vi "Configure_Filters.vi"(7 "I2C Channel":u8, 8 "error in (no error)":errorcluster, 9 "Filtered Data Selection":T1(ring), 10 "High-Pass Cutoff Frequency":T2(ring), 11 "LINX Resource In":T3) -> (0 "error out":errorcluster, 3 "LINX Resource Out":T3)   [LabVIEW 2014, in "LMH-LINX.lvlib" / "LIS331HH.lvlib"]
doc: "This VI ebales and configures High-Pass output filters and Enables/Disables Filter bypass. \nLow Pass filters and cutoff frequency is based of Output Data Rate (ORD) set with Initialize.vi and Set_ODR.vi\n\n**Author: Stas Legedza"
uses:
  <vilib>/MakerHub/LINX/Public/Sensors/Accelerometer/LIS331HH/LIS331HH.lvlib
  <vilib>/MakerHub/LINX/Private/Type Defs/LINX Ref.ctl
  <vilib>/MakerHub/LINX/Private/Type Defs/Platform.ctl
  <vilib>/MakerHub/LINX/Private/Type Defs/Interface.ctl
  <vilib>/MakerHub/LINX/Private/Device/Type Defs/LINX Device Config.ctl
  <vilib>/MakerHub/LINX/Private/Device/Type Defs/TCP Config.ctl
  <vilib>/MakerHub/LINX/Private/Device/Type Defs/Channels.ctl
  <vilib>/MakerHub/LINX/Private/Local IO/LinxI2cWrite.vi
  <vilib>/MakerHub/LINX/Public/Utilities/Check Channel.vi
  <vilib>/MakerHub/LINX/Private/Utilties/Generate Error.vi
  <vilib>/MakerHub/LINX/LMH-LINX.lvlib
  <vilib>/MakerHub/LINX/Private/Device/Device.lvlib
panel:
  # "NOTE: LP Cutoff is based on a Output \nData Rate (ODR) settings\ni.e. @ODR of 50 Hz, LP_cutoff  is 37 Hz"
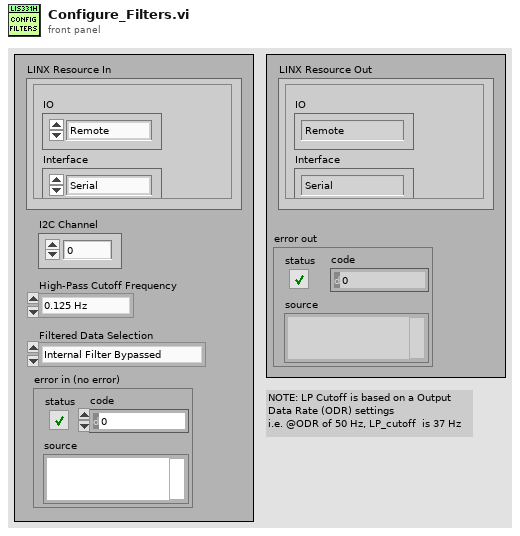
[diagram p1: front panel]
types:
  T1 = enum16{"Internal Filter Bypassed", "Data via Internal Filter"}
  T2 = enum16{"0.125 Hz", "0.25 Hz", "0.5 Hz", "1 Hz", "2 Hz", "2.5 Hz", "4 Hz", "5 Hz", "8 Hz", "10 Hz", "20 Hz"}
  T3 = typedef "LMH-LINX.lvlib/LINX Ref.ctl" = cluster{"IO":T4, "Interface":T5, "LINX Device Config":T6}
  T4 = typedef "LMH-LINX.lvlib/Platform.ctl" = enum16{"Remote", "Local"}
  T5 = typedef "LMH-LINX.lvlib/Interface.ctl" = enum16{"Serial", "TCP"}
  T6 = typedef "LMH-LINX.lvlib/Device.lvlib/LINX Device Config.ctl" = cluster{"Interface":T5, "COM Port":refnum<visa-resource-name>, "TCP Configuration":T7, "Device Family":u8, "Device ID":u8, "Device Name":string, "TCP Ref":refnum<k5>, "Channels":T8}
  T7 = typedef "LMH-LINX.lvlib/Device.lvlib/TCP Config.ctl" = cluster{"IP Address":string, "Port":u16}
  T8 = typedef "LMH-LINX.lvlib/Channels.ctl" = cluster{"DI":u8[], "DO":u8[], "AI":u8[], "AO":u8[], "PWM":u8[], "QE":u8[], "UART":u8[], "I2C 2":u8[], "SPI":u8[], "CAN":u8[], "Servo":u8[], "AI Ref (V)":dbl, "AI Resolution (Bits)":u8, "AO Ref (V)":dbl, "AO Resolution (Bits)":u8}
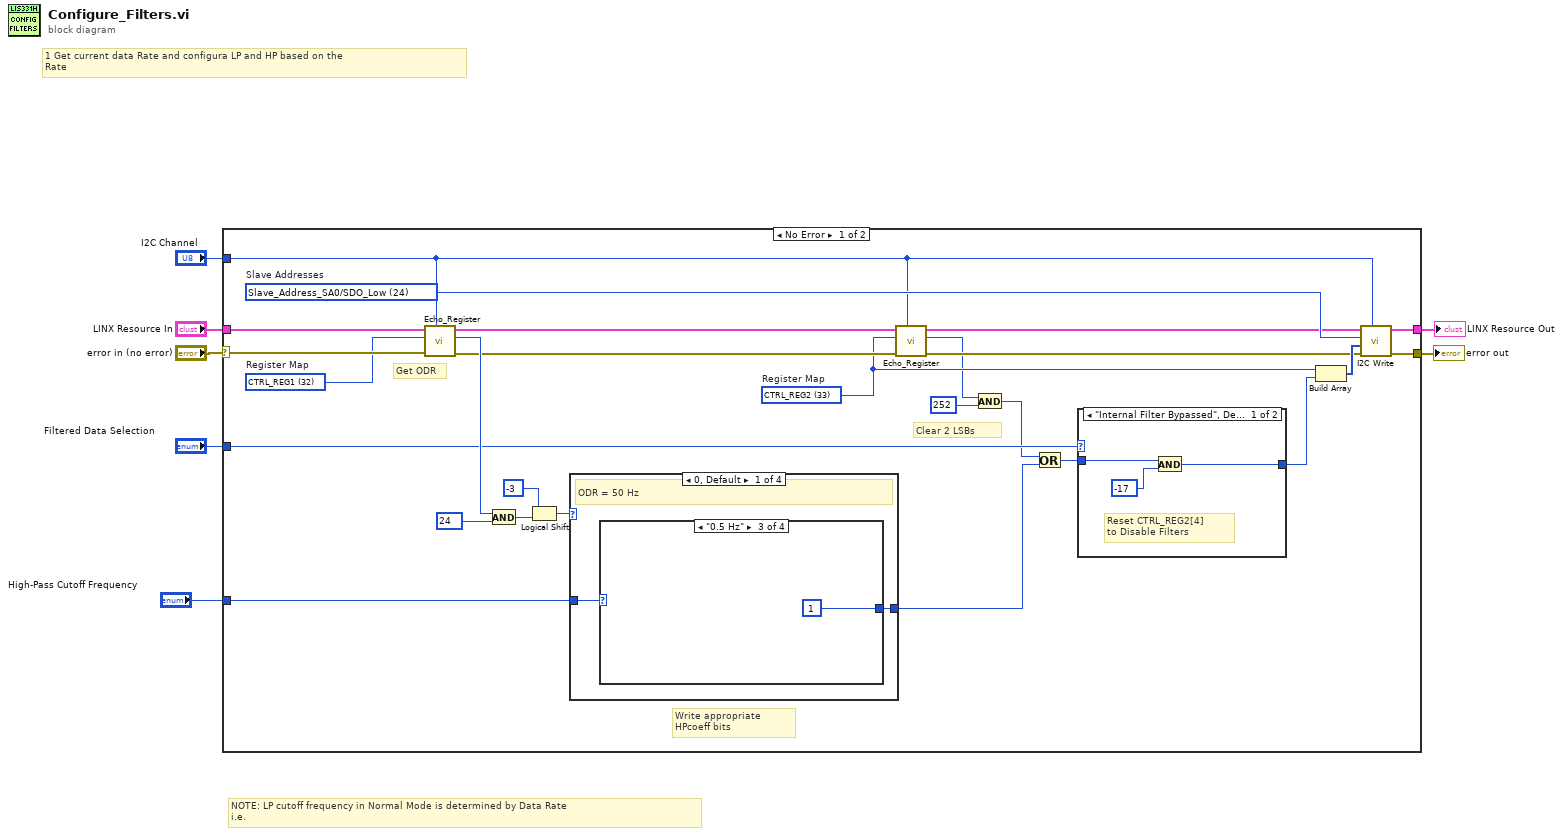
[diagram p0: block diagram]
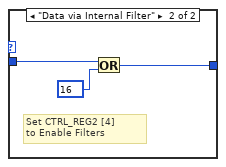
[diagram p2: hidden frame]
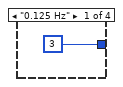
[diagram p3: hidden frame]
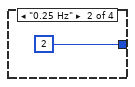
[diagram p4: hidden frame]
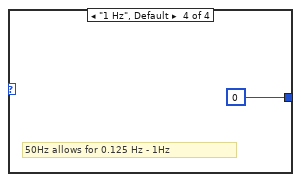
[diagram p5: hidden frame]
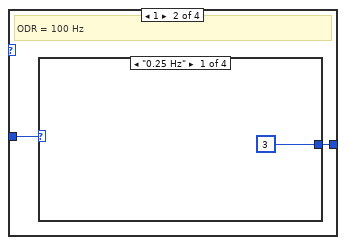
[diagram p6: hidden frame]
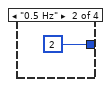
[diagram p7: hidden frame]
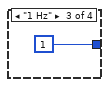
[diagram p8: hidden frame]
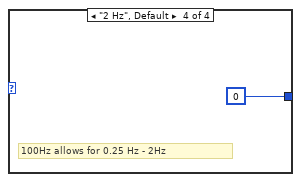
[diagram p9: hidden frame]
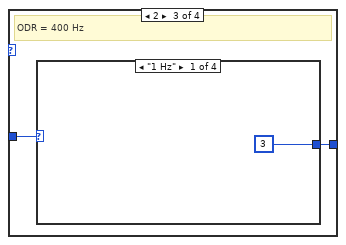
[diagram p10: hidden frame]
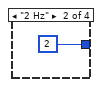
[diagram p11: hidden frame]
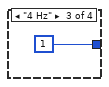
[diagram p12: hidden frame]
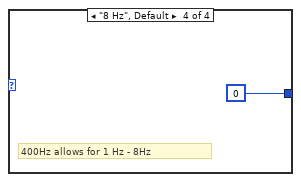
[diagram p13: hidden frame]
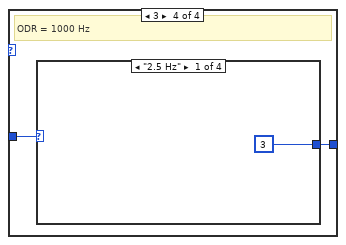
[diagram p14: hidden frame]
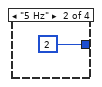
[diagram p15: hidden frame]
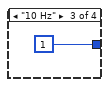
[diagram p16: hidden frame]
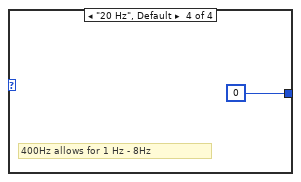
[diagram p17: hidden frame]
diagram:
  # "NOTE: LP cutoff frequency in Normal Mode is determined by Data Rate\ni.e."
  # "1 Get current data Rate and configura LP and HP based on the\nRate"
  n1 = case shown="No Error" "error in (no error)" {
    selector: "error in (no error)" -> [w29 w65]
    tunnel: [w32 w65] -> w6
    tunnel: "LINX Resource In" -> [w30 w64]
    tunnel: "I2C Channel" -> [w22 _]
    tunnel: [w31 w64] -> w3
    tunnel: "High-Pass Cutoff Frequency" -> [w25 _]
    tunnel: "Filtered Data Selection" -> [w12 _]
    frame No Error {
      w19 = u8 33 items=["CTRL_REG1"=32, "CTRL_REG2"=33, "CTRL_REG3"=34, "CTRL_REG4"=35, "CTRL_REG5"=36, "HP_FILTER_RESET"=37, "REFERENCE"=38, "STATUS_REG"=39, "OUT_X_L"=40, "OUT_X_H"=41, "OUT_Y_L"=42, "OUT_Y_H"=43, "OUT_Z_L"=44, "OUT_Z_H"=45, "INT1_CFG"=48, "INT1_SOURCE"=49, "INT1_THS"=50, "INT1_DURATION"=51, "INT2_CFG"=52, "INT2_SOURCE"=53, "INT2_THS"=54, "INT2_DURATION"=55]  # Register Map
      w18 = u8 32 items=["CTRL_REG1"=32, "CTRL_REG2"=33, "CTRL_REG3"=34, "CTRL_REG4"=35, "CTRL_REG5"=36, "HP_FILTER_RESET"=37, "REFERENCE"=38, "STATUS_REG"=39, "OUT_X_L"=40, "OUT_X_H"=41, "OUT_Y_L"=42, "OUT_Y_H"=43, "OUT_Z_L"=44, "OUT_Z_H"=45, "INT1_CFG"=48, "INT1_SOURCE"=49, "INT1_THS"=50, "INT1_DURATION"=51, "INT2_CFG"=52, "INT2_SOURCE"=53, "INT2_THS"=54, "INT2_DURATION"=55]  # Register Map
      w33 = u8 24 items=["Slave_Address_SA0/SDO_Low"=24, "Slave_Address_SA0/SDO_High"=25]  # Slave Addresses
      # "Write appropriate\nHPcoeff bits"
      # "Clear 2 LSBs"
      # "Get ODR"
      n2 = call <vilib>:"Echo_Register.vi"("I2C Channel"=w22, "error in (no error)"=w29, "Register to Echo"=w18, "LINX Resource In"=w30) -> ("error out"=w23:errorcluster, "Register Word"=w27:u8, "LINX Resource Out"=w24:T3)  [unwired: 5 in]
      n3 = And(x=w27, y=u8 24) -> (x .and. y?=w17:u8)
      n4 = Logical Shift(y=i16 -3, x=w17) -> (x << y=w16:u8)
      n5 = case shown="0, Default" w16 {
        tunnel: w25 -> [w41 w47 w53 w59]
        tunnel: [w40 w46 w52 w58] -> w10
        frame 0, Default {
          # "ODR = 50 Hz"
          n6 = case shown="\"0.5 Hz\"" w41 {
            tunnel: [u8 3 ("y") u8 2 ("y") u8 1 ("y") u8 0 ("y")] -> w40
            frame "0.125 Hz" {
            }
            frame "0.25 Hz" {
            }
            frame "0.5 Hz" {
            }
            frame "1 Hz", Default {
              # "50Hz allows for 0.125 Hz - 1Hz"
            }
          }
        }
        frame 1 {
          # "ODR = 100 Hz"
          n7 = case shown="\"0.25 Hz\"" w47 {
            tunnel: [u8 3 ("y") u8 2 ("y") u8 1 ("y") u8 0 ("y")] -> w46
            frame "0.25 Hz" {
            }
            frame "0.5 Hz" {
            }
            frame "1 Hz" {
            }
            frame "2 Hz", Default {
              # "100Hz allows for 0.25 Hz - 2Hz"
            }
          }
        }
        frame 2 {
          # "ODR = 400 Hz"
          n8 = case shown="\"1 Hz\"" w53 {
            tunnel: [u8 3 ("y") u8 2 ("y") u8 1 ("y") u8 0 ("y")] -> w52
            frame "1 Hz" {
            }
            frame "2 Hz" {
            }
            frame "4 Hz" {
            }
            frame "8 Hz", Default {
              # "400Hz allows for 1 Hz - 8Hz"
            }
          }
        }
        frame 3 {
          # "ODR = 1000 Hz"
          n9 = case shown="\"2.5 Hz\"" w59 {
            tunnel: [u8 3 ("y") u8 2 ("y") u8 1 ("y") u8 0 ("y")] -> w58
            frame "2.5 Hz" {
            }
            frame "5 Hz" {
            }
            frame "10 Hz" {
            }
            frame "20 Hz", Default {
              # "400Hz allows for 1 Hz - 8Hz"
            }
          }
        }
      }
      n10 = call <vilib>:"Echo_Register.vi"("I2C Channel"=w22, "error in (no error)"=w23, "Register to Echo"=w19, "LINX Resource In"=w24) -> ("error out"=w20:errorcluster, "Register Word"=w13:u8, "LINX Resource Out"=w21:T3)  [unwired: 5 in]
      n11 = And(x=w13, y=u8 252) -> (x .and. y?=w11:u8)
      n12 = Or(x=w11, y=w10) -> (x .or. y?=w9:u8)
      n13 = case shown="\"Internal Filter Bypassed\", Default" w12 {
        tunnel: w9 -> [w36 w39]
        tunnel: [w35 w37] -> w8
        frame "Internal Filter Bypassed", Default {
          # "Reset CTRL_REG2[4]\nto Disable Filters"
          n14 = And(x=w36, y=i8 -17) -> (x .and. y?=w35:u8)
        }
        frame "Data via Internal Filter" {
          # "Set CTRL_REG2 [4]\nto Enable Filters"
          n15 = Or(x=w39, y=u8 16) -> (x .or. y?=w37:u8)
        }
      }
      n16 = Build Array(w19, w8) -> (w28:u8[])
      n17 = call <vilib>:"I2C Write.vi"("I2C Channel"=w22, "Error In"=w20, "Data"=w28, "I2C Slave Address (0)"=w33, "LINX Resource"=w21) -> ("Error Out"=w32:errorcluster, "LINX Resource"=w31:T3)  [unwired: 5 in]
    }
    frame Error {
    }
  }
  "error out" <- w6
  "LINX Resource Out" <- w3
